vi "NXTLineLeader-DM.vi"(0 "Input of NXTLineLeader":T2={"Base Power"=75, "Base Direction"=FALSE, "Operation"=enum."Track Line"} {"Base Power" min=0 max=100}, 2 "NXT":T4={"error"={"status"=FALSE, "code"=0, "source"=""}, "address"="", "NXT #"=0, "Show Error"=FALSE, "Connection"=4} {"Connection" items=["USB", "Bluetooth", "USB then Bluetooth", "Last Connection", "Preference"]}, 3 "Input Port":T3 items=["Port 1", "Port 2", "Port 3", "Port 4"]) -> (1 "Output of NXTLineLeader":T1, 4 "NXT dup":T4={"error"={"status"=FALSE, "code"=0, "source"=""}, "address"="", "NXT #"=0, "Show Error"=FALSE, "Connection"=4} caption="NXT" {"Connection" items=["USB", "Bluetooth", "USB then Bluetooth", "Last Connection", "Preference"]})   [LabVIEW 2009]
doc: "This vi will allow yout to track a line given its inputs and allows you to change the PID to perfect your NXT's line tracking based on its design."
uses:
  <vilib>/NXT/Subs/LVHSConnector.ctl
  <vilib>/NXT/Block Support/NXT_InputPort.ctl
  <vilib>/NXT/Block Support/HWPage.SensorType.ctl
  <vilib>/NXT/Block Support/HWPage.SensorMode.ctl
panel:
  out "Base Direction":bool
  out "Base Power":i8
  out "Boolean":bool caption="Yes / No"
  in  "Steering":i8=5
  out "Status":bool
  out "Average":i8 caption="Line Data"
  out "Motor 2 Power":u8=93
  out "Motor 1 Power":u8=57
  out "Motor 2 direction":bool=TRUE
  out "Motor 1 direction":bool=TRUE
  # "NXT_InputPort.ctlmindsensors.com\nCopyright (c) 2009 by mindsensors.com\nEmail: info (<at>) mindsensors (<dot>) com\n\nThis program is free software. You can redistribute it and/or modify\nit under the terms of the GNU General Public License as published by\nthe Free Software Foundation; version 3 of the License.\nRead the license at: http://www.gnu.org/licenses/gpl.txt"
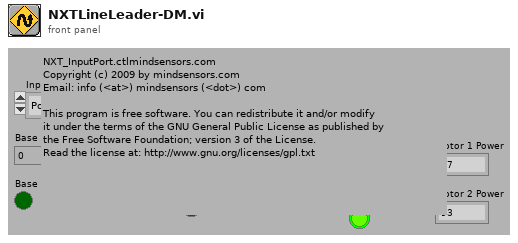
[diagram p1: front panel]
types:
  T1 = cluster{"Average":u8, "Steering":i8, "Base Direction":bool, "Base Power":i8, "Motor 1 Direction":bool, "Motor 1 Power":i32, "Motor 2 Direction":bool, "Motor 2 Power":i32, "Success?":bool}
  T2 = cluster{"Base Power":i8, "Base Direction":bool, "Operation":enum32{"Track Line", "Read Raw Sensor ", "Read Sensor Avg"}}
  T3 = typedef "NXT_InputPort.ctl" = u8
  T4 = typedef "LVHSConnector.ctl" = cluster{"error":errorcluster, "address":string, "NXT #":i32, "Show Error":bool, "Connection":u16}
  T5 = typedef "HWPage.SensorType.ctl" = u8
  T6 = typedef "HWPage.SensorMode.ctl" = u8
  T7 = enum32{"Track Line", "Read Raw Sensor ", "Read Sensor Avg"}
  T8 = cluster{u8, "Steering":i8, "Base Direction":bool, "Base Power":i8, bool, "Numeric Out":i32, bool, "Numeric Out":i32, "Success?":bool}
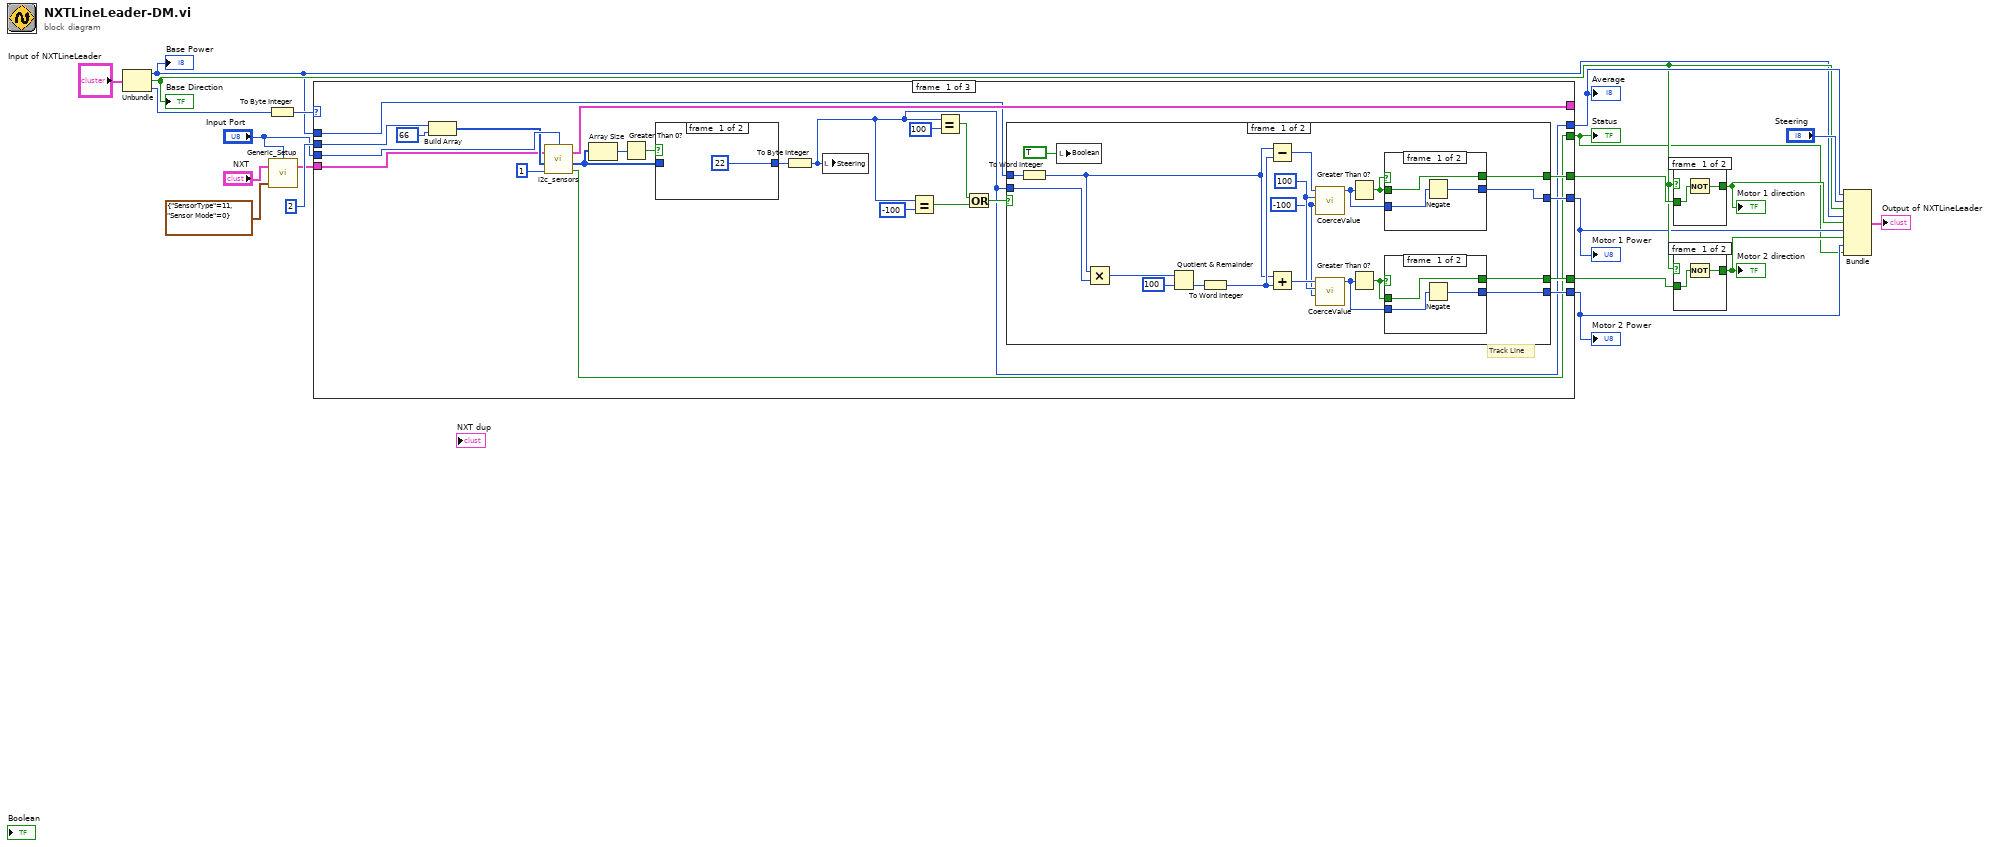
[diagram p0: block diagram]
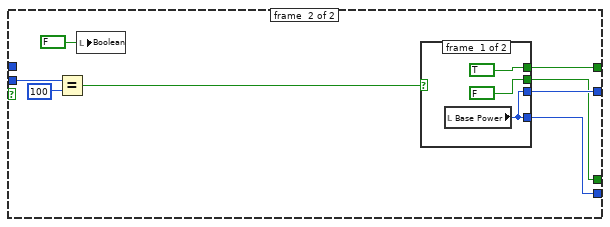
[diagram p4: hidden frame]
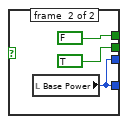
[diagram p5: hidden frame]
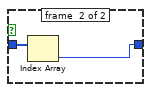
[diagram p6: hidden frame]
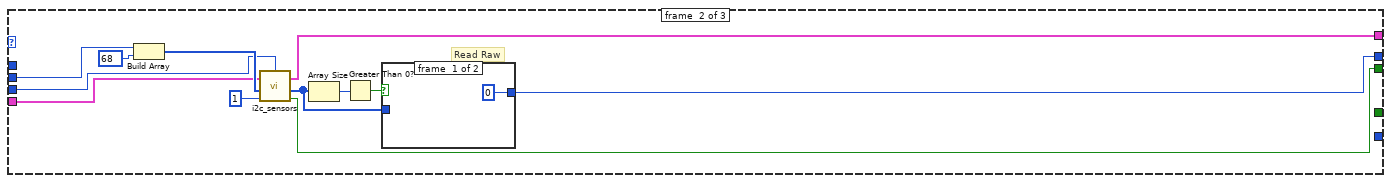
[diagram p7: hidden frame]
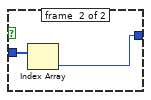
[diagram p8: hidden frame]
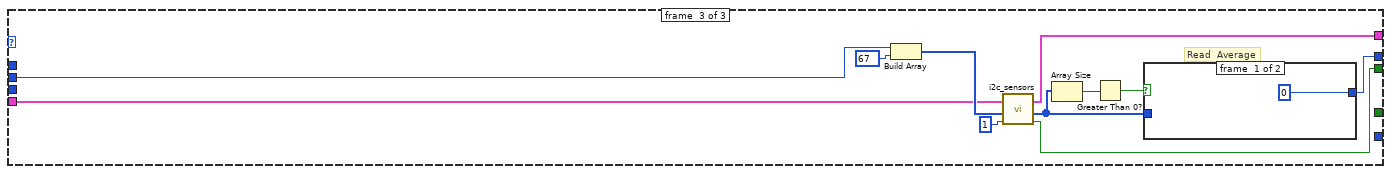
[diagram p9: hidden frame]
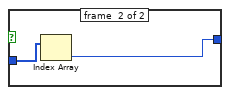
[diagram p10: hidden frame]
diagram:
  n1 = Unbundle("Input of NXTLineLeader") -> ("Base Power"=w7:i8, "Base Direction"=w8:bool, "Operation"=w11:T7)
  "Base Power" <- w7
  "Base Direction" <- w8
  n2 = To Byte Integer(number=w11) -> (8bit integer=w15:i8)
  n3 = call <vilib>:"Generic_Setup.vi"("Sensor Setup"=cluster{"SensorType":T5, "Sensor Mode":T6} {"SensorType"=11, "Sensor Mode"=0}, "NXT"="NXT", "Port"="Input Port") -> ("NXT"=w12:T4)  [unwired: 1 out]
  n4 = case shown="0, Default" w15 {
    tunnel: 2 -> [w27 w99 w110]
    tunnel: [w32 w102 w116] -> w10
    tunnel: [w42 _ _] -> w5
    tunnel: [w41 _ _] -> w16
    tunnel: [w40 _ _] -> w17
    tunnel: [w39 _ _] -> w3
    tunnel: [w28 w96 w112] -> w2
    tunnel: "Input Port" -> [w31 w91 _]
    tunnel: w12 -> [w22 w93 w106]
    tunnel: [w23 w92 w107] -> _
    tunnel: w7 -> [w21 _ _]
    frame #0 {
      # "Track Line"
      n5 = Build Array(w27, u8 66 ("register")) -> (w30:i32[])
      n6 = call <vilib>:"i2c_sensors.vi"("Return Length"=u8 1 ("ReturnLength"), "Bytes to Write"=w30, "NXT"=w22, "Port"=w31) -> ("Success?"=w28:bool, "Bytes read"=w24:u8[], "NXT"=w23:T4)  [unwired: 1 in]
      n7 = Array Size(array=w24) -> (size(s)=w25:i32)
      n8 = Greater Than 0?(x=w25) -> (x > 0?=w43:bool)
      n9 = case shown="True" w43 {
        tunnel: w24 -> [_ w90]
        tunnel: [u8 22 w89] -> w34
        frame #0 {
        }
        frame #1 {
          n10 = Index Array(array=w90) -> (element=w89:u8)  [unwired: 1 in]
        }
      }
      n11 = To Byte Integer(number=w34) -> (8bit integer=w32:i8)
      n12 = local write "Steering"(w32) -> ()
      n13 = Equal?(x=w32, y=-100) -> (x = y?=w35:bool)
      n14 = Equal?(x=w32, y=100) -> (x = y?=w36:bool)
      n15 = Or(x=w36, y=w35) -> (x .or. y?=w33:bool)
      n16 = case shown="True" w33 {
        tunnel: [w62 w77] -> w42
        tunnel: [w61 w76] -> w41
        tunnel: [w58 w75] -> w40
        tunnel: [w57 w78] -> w39
        tunnel: w32 -> [w49 w80]
        tunnel: w21 -> [w44 _]
        frame #0 {
          w51 = i16 -100 ("lower limit")
          w52 = i16 100 ("upper limit")
          n17 = To Word Integer(number=w44) -> (16bit integer=w48:i16)
          n18 = local write "Boolean"(TRUE ("Boolean")) -> ()
          n19 = Multiply(x=w48, y=w49) -> (x*y=w47:i16)
          n20 = Quotient & Remainder(x=w47, y=i16 100) -> (floor(x/y)=w45:i16)  [unwired: 1 out]
          n21 = To Word Integer(number=w45) -> (16bit integer=w63:i16)
          n22 = Subtract(x=w48, y=w63) -> (x-y=w55:i16)
          n23 = Add(x=w48, y=w63) -> (x+y=w53:i16)
          n24 = call <vilib>:"CoerceValue.vi"("Min (0)"=w51, "Max (100)"=w52, "Numeric"=w55) -> ("Numeric Out"=w56:i32)  [unwired: 8 in]
          n25 = call <vilib>:"CoerceValue.vi"("Min (0)"=w51, "Max (100)"=w52, "Numeric"=w53) -> ("Numeric Out"=w54:i32)  [unwired: 8 in]
          n26 = Greater Than 0?(x=w56) -> (x > 0?=w60:bool)
          n27 = Greater Than 0?(x=w54) -> (x > 0?=w59:bool)
          n28 = case shown="True" w60 {
            tunnel: [w71 w72] -> w62
            tunnel: [w70 w73] -> w61
            tunnel: w60 -> [w70 w73]
            tunnel: w56 -> [w69 w72]
            frame #0 {
              n29 = Negate(x=w69) -> (-x=w71:i32)
            }
            frame #1 {
            }
          }
          n30 = case shown="True" w59 {
            tunnel: [w66 w67] -> w57
            tunnel: [w65 w68] -> w58
            tunnel: w59 -> [w65 w68]
            tunnel: w54 -> [w64 w67]
            frame #0 {
              n31 = Negate(x=w64) -> (-x=w66:i32)
            }
            frame #1 {
            }
          }
        }
        frame #1 {
          n32 = Equal?(x=w80, y=100) -> (x = y?=w79:bool)
          n33 = local write "Boolean"(FALSE ("Boolean")) -> ()
          n34 = case shown="False" w79 {
            tunnel: [w84 w86] -> w77
            tunnel: [TRUE FALSE] -> w76
            tunnel: [w84 w86] -> w78
            tunnel: [FALSE TRUE] -> w75
            frame #0 {
              n35 = local read "Base Power"() -> (w84:i8)
            }
            frame #1 {
              n36 = local read "Base Power"() -> (w86:i8)
            }
          }
        }
      }
    }
    frame #1 {
      # "Read Raw"
      n37 = Build Array(w99, u8 68 ("register")) -> (w97:i32[])
      n38 = call <vilib>:"i2c_sensors.vi"("Return Length"=u8 1 ("ReturnLength"), "Bytes to Write"=w97, "NXT"=w93, "Port"=w91) -> ("Success?"=w96:bool, "Bytes read"=w94:u8[], "NXT"=w92:T4)  [unwired: 1 in]
      n39 = Array Size(array=w94) -> (size(s)=w95:i32)
      n40 = Greater Than 0?(x=w95) -> (x > 0?=w101:bool)
      n41 = case shown="True" w101 {
        tunnel: w94 -> [_ w105]
        tunnel: [u8 0 w104] -> w102
        frame #0 {
        }
        frame #1 {
          n42 = Index Array(array=w105) -> (element=w104:u8)  [unwired: 1 in]
        }
      }
    }
    frame #2 {
      # "Read  Average"
      n43 = Build Array(w110, u8 67 ("register")) -> (w111:i32[])
      n44 = call <vilib>:"i2c_sensors.vi"("Return Length"=u8 1 ("ReturnLength"), "Bytes to Write"=w111, "NXT"=w106) -> ("Success?"=w112:bool, "Bytes read"=w113:u8[], "NXT"=w107:T4)  [unwired: 2 in]
      n45 = Array Size(array=w113) -> (size(s)=w114:i32)
      n46 = Greater Than 0?(x=w114) -> (x > 0?=w115:bool)
      n47 = case shown="True" w115 {
        tunnel: w113 -> [_ w119]
        tunnel: [u8 0 w118] -> w116
        frame #0 {
        }
        frame #1 {
          n48 = Index Array(array=w119) -> (element=w118:u8)  [unwired: 1 in]
        }
      }
    }
  }
  "Motor 1 Power" <- w5
  "Motor 2 Power" <- w3
  "Average" <- w10
  "Status" <- w2
  n49 = case shown="False" w8 {
    tunnel: w16 -> [w121 w122]
    tunnel: [w120 w122] -> w6
    frame #0 {
      n50 = Not(x=w121) -> (.not. x?=w120:bool)
    }
    frame #1 {
    }
  }
  "Motor 1 direction" <- w6
  n51 = case shown="False" w8 {
    tunnel: w17 -> [w124 w125]
    tunnel: [w123 w125] -> w4
    frame #0 {
      n52 = Not(x=w124) -> (.not. x?=w123:bool)
    }
    frame #1 {
    }
  }
  "Motor 2 direction" <- w4
  n53 = Bundle(w10, "Steering"="Steering", "Base Direction"=w8, "Base Power"=w7, w6, "Numeric Out"=w5, w4, "Numeric Out"=w3, "Success?"=w2) -> (→"Output of NXTLineLeader":T8)  [unwired: 1 in]
